vi "Actor Core.vi"(8 "error in":errorcluster, 11 "UIA_ChildTestMaster in":refnum<class "UIA_UTsupport.lvclass">) -> (0 "error out":errorcluster, 3 "Actor out":refnum<class "Actor.lvclass">)   [LabVIEW 2020, in "UIA_UTsupport.lvlib" / "UIA_UTsupport.lvclass"]
doc: "(<B>Filename</B>: Actor Framework.lvlib:Actor.lvclass:Actor Core.vi)\n\nReceives messages to the actor, reacts to them, and initiates any error handling that may shut the actor down.\n\nDescendant classes may override this VI to append parallel tasks for the actor to complete while it handles messages. Overrides use the Call Parent Method node."
uses:
  UIA_UTsupport.lvclass
  support/Actor Framework.lvlibp/1abvi3w/vi.lib/ActorFramework/Actor/Actor.lvclass
  UI_Actor/UI_Actor Messages/UI_ShowIn_FreeWindow Msg/UI_ShowIn_FreeWindow Msg.lvclass/UI_ShowIn_FreeWindow Msg.ctl
  support/Actor Framework.lvlibp/1abvi3w/vi.lib/ActorFramework/Message Enqueuer/Enqueue.vi
  UI_Actor/UI_Actor Messages/UI_ShowIn_FreeWindow Msg/UI_ShowIn_FreeWindow Msg.lvclass
  UI_Actor/UI_Actor/UI_Actor.lvclass
panel:
  out "S2.indic":dbl caption="Ctl1"
  out "S1.Ctl1":dbl caption="Ctl1"
  # "UI ACTOR Unit test support"
  # "Je suis dispo pour les UT avec mes gloglo super nickel"
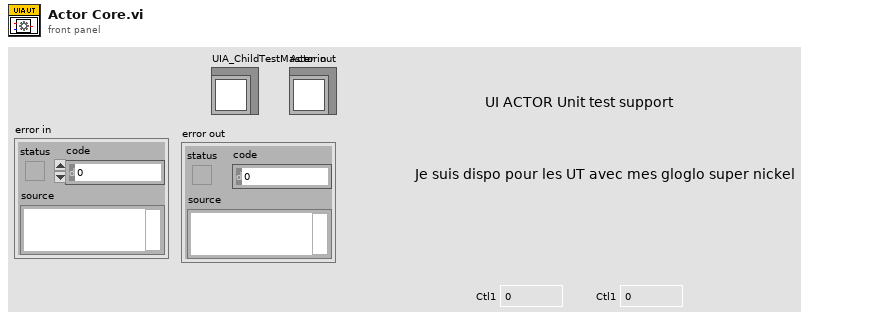
[diagram p1: front panel]
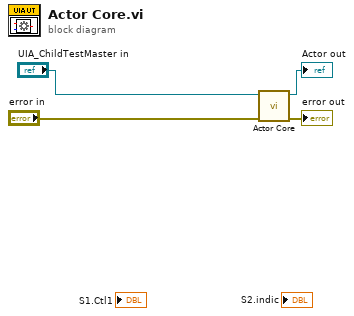
[diagram p0: block diagram]
diagram:
  n1 = call-parent "Actor Core.vi"("error in"="error in", "UI_Actor in"="UIA_ChildTestMaster in") -> ("error out"=→"error out":errorcluster, "Actor out"=→"Actor out":refnum<class "Actor.lvclass">)  [unwired: 8 in]
